vi "Create New Group.vi"(8 "error in (no error)":errorcluster, 11 "Selector in":refnum<class "Selector.lvclass">) -> (0 "error out":errorcluster, 3 "Selector out":refnum<class "Selector.lvclass">)   [LabVIEW 2019, in "Selector.lvclass"]
uses:
  Selector.lvclass
  Selector.lvclass/Selector.ctl
  cce5df9e-5964-4f11-9dff-719ececaf2a4.vi
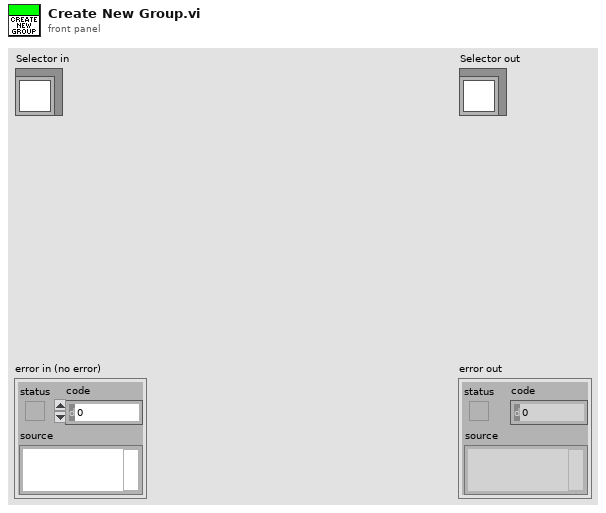
[diagram p1: front panel]
types:
  T1 = cluster{"Name":string, "Group":string, "Enabled":bool}[]
  T2 = cluster{"Name":string, "Group":string, "Enabled":bool}
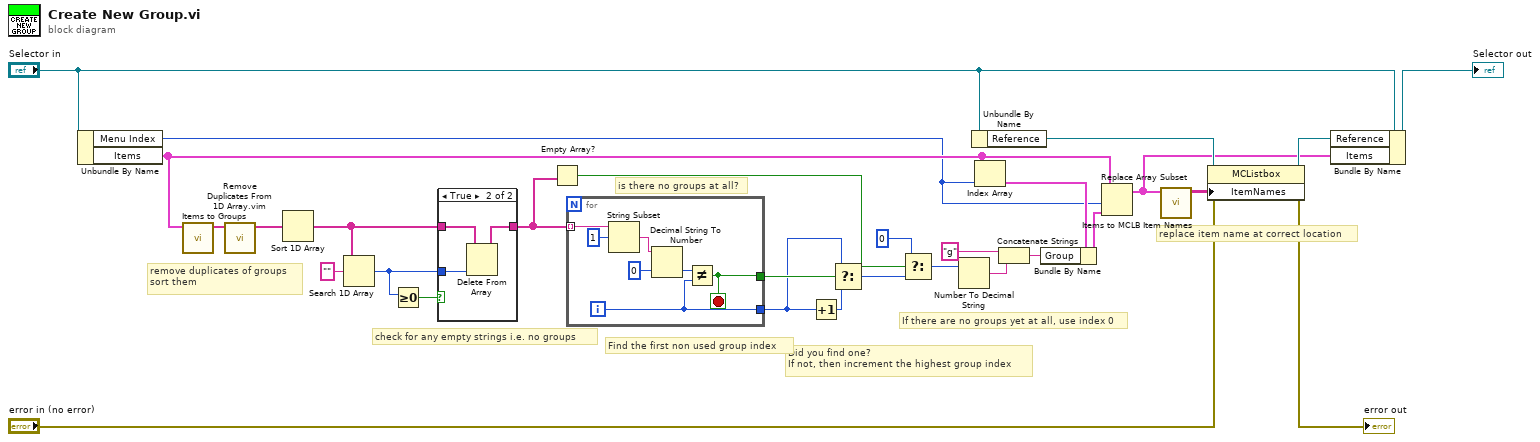
[diagram p0: block diagram]
diagram:
  # "replace item name at correct location"
  # "If there are no groups yet at all, use index 0"
  # "Did you find one?\nIf not, then increment the highest group index"
  # "Find the first non used group index"
  # "is there no groups at all?"
  # "check for any empty strings i.e. no groups"
  # "remove duplicates of groups\nsort them"
  n1 = Unbundle By Name("Selector in") -> ("Menu Index"=w1:i32, "Items"=w2:T1)
  n2 = call "Items to Groups.vi"("Items"=w2) -> ("Groups"=w8:string[])  [unwired: 6 in]
  n3 = call "Remove Duplicates From 1D Array.vim"("array"=w8) -> ("array with duplicates removed"=w29:string[])  [unwired: 10 in]
  n4 = Sort 1D Array(array=w29) -> (sorted array=w19:string[])
  n5 = Search 1D Array(1D array=w19, element="") -> (index of element=w26:i32)  [unwired: 1 in]
  n6 = Greater Or Equal To 0?(x=w26) -> (x >= 0?=w27:bool)
  n7 = case shown="True" w27 {
    tunnel: w19 -> [w30 w33]
    tunnel: [w30 w32] -> w21
    tunnel: w26 -> [_ w31]
    frame False {
    }
    frame True {
      n8 = Delete From Array(array=w33, index=w31) -> (array with subset deleted=w32:string[])  [unwired: 1 in, 1 out]
    }
  }
  n9 = Empty Array?(array=w21) -> (empty?=w13:bool)
  n10 = for {
    tunnel: w21 -> [w35] mode=indexing
    tunnel: [w37] -> w25
    tunnel: [w34] -> w17
    i -> [w34]
    stop <- w37 stop-if-true
    n11 = String Subset(string=w35, offset (0)=1) -> (substring=w36:string)  [unwired: 1 in]
    n12 = Decimal String To Number(string=w36, default (0L)=0) -> (number=w38:i32)  [unwired: 1 in, 1 out]
    n13 = Not Equal?(x=w38, y=w34) -> (x != y?=w37:bool)
  }
  n14 = Increment(x=w17) -> (x+1=w18:i32)
  n15 = Select(t=w17, s=w25, f=w18) -> (s? t:f=w15:i32)
  n16 = Select(t=0, s=w13, f=w15) -> (s? t:f=w20:i32)
  n17 = Number To Decimal String(number=w20) -> (decimal integer string=w16:string)  [unwired: 1 in]
  n18 = Unbundle By Name("Selector in") -> ("Reference"=w23:refnum<vi>)
  n19 = Index Array(array=w2, index=w1) -> (element=w7:T2)
  n20 = Concatenate Strings("g" ("string"), w16) -> (w6:string)
  n21 = Bundle By Name(cluster=w7, "Group"=w6) -> (w3:T2)
  n22 = Replace Array Subset(array=w2, new element=w3, index=w1) -> (w4:T1)
  n23 = call "Items to MCLB Item Names.vi"("Items"=w4) -> ("Item Names"=w5:string[][])  [unwired: 6 in]
  n24 = property class="MCListbox"(reference=w23, error in="error in (no error)", "ItemNames"=w5) -> (reference out=w12:refnum<vi>, error out=→"error out":errorcluster)
  n25 = Bundle By Name(cluster="Selector in", "Reference"=w12, "Items"=w4) -> (→"Selector out":refnum<class "Selector.lvclass">)
